vi "FFT_ADXL345.vi"() -> ()   [LabVIEW 2015]
uses:
  <vilib>/Utility/error.llb/DialogType.ctl
  <vilib>/Instr/_visa.llb/VISA Configure Serial Port (Instr).vi
panel:
  in  "Frame rate":i32
  out "FFT Graph":dbl[](graph)
  out "TIME Graph":dbl[](graph)
  out "Z":dbl
  out "Y":dbl
  out "X":dbl
  out "acceleretion(m/s^2)":cluster{"X":dbl, "Y":dbl, "Z":dbl}
  out "Waveform Chart":u32(graph)
  out "1LOOP(ms)":u32
  in  "FFT SIZE":i32
  out "DATA array":dbl[](array[numeric])
  in  "Axis":enum16{"Z", "Y", "X"}(ring)
  in  "DAC":i32
  out "DATA":string
  out "DATA LENGHT":i32
  out "Z":string
  out "Y":string
  out "X":string
  out "X(mg)":dbl format="%.2f"
  out "Y(mg)":dbl format="%.2f"
  out "Z(mg)":dbl format="%.2f"
  out "Akselerasi (mg)":dynamicdata(graph)
  in  "stop":bool
  in  "VISA RESOURCE":refnum<visa-resource-name>="COM4"
  out "millisecond timer value":u32
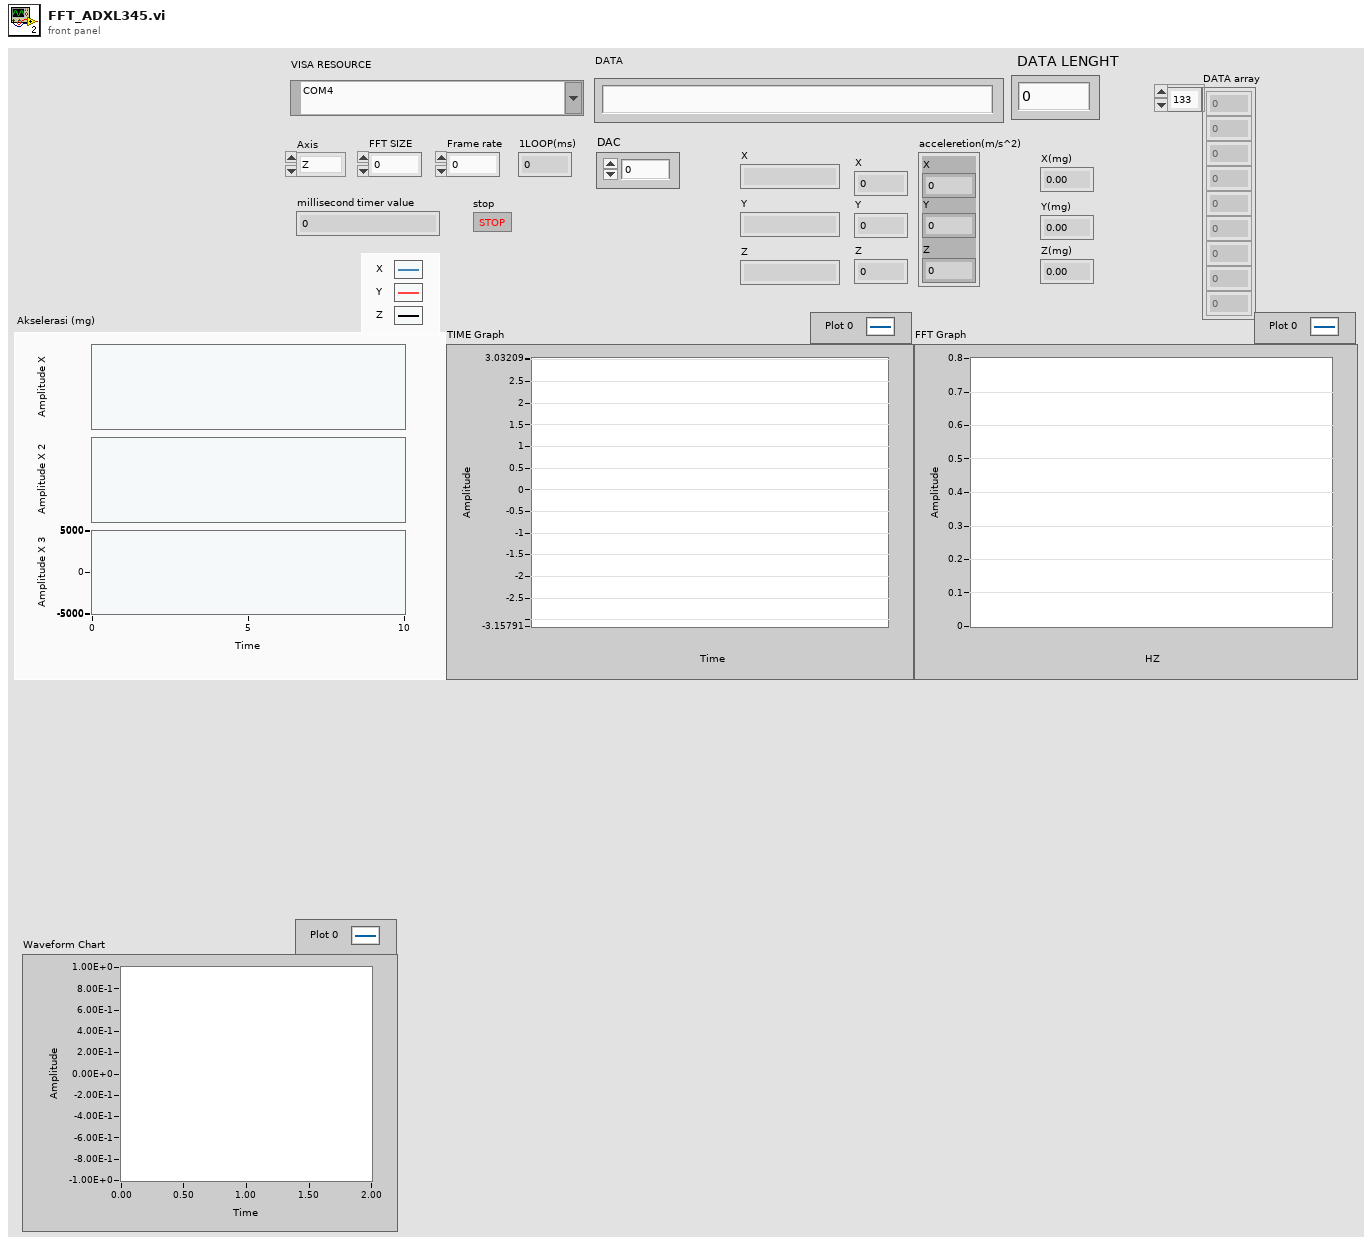
[diagram p1: front panel]
types:
  T1 = typedef "DialogType.ctl" = u16
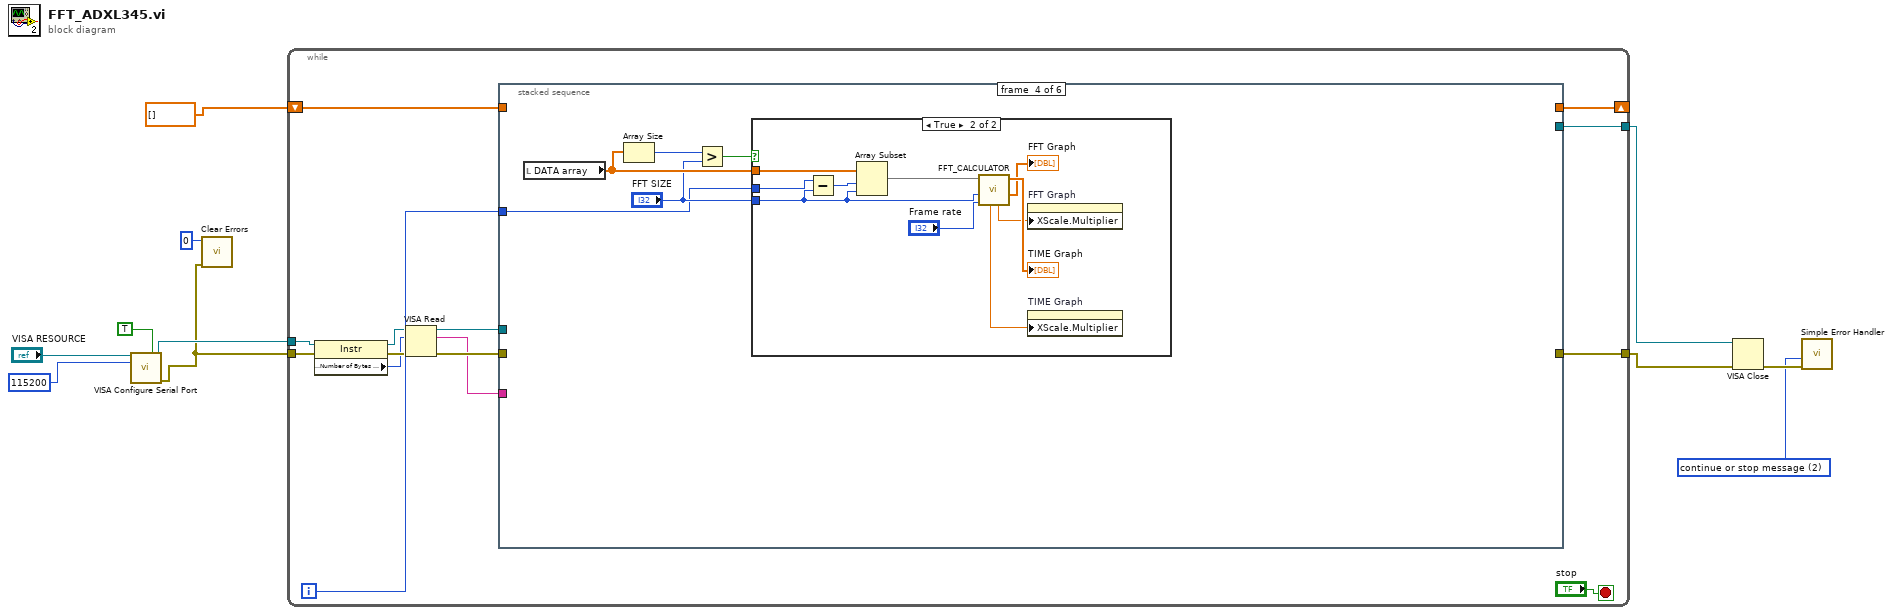
[diagram p0: block diagram]
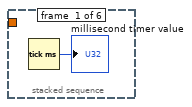
[diagram p2: hidden frame]
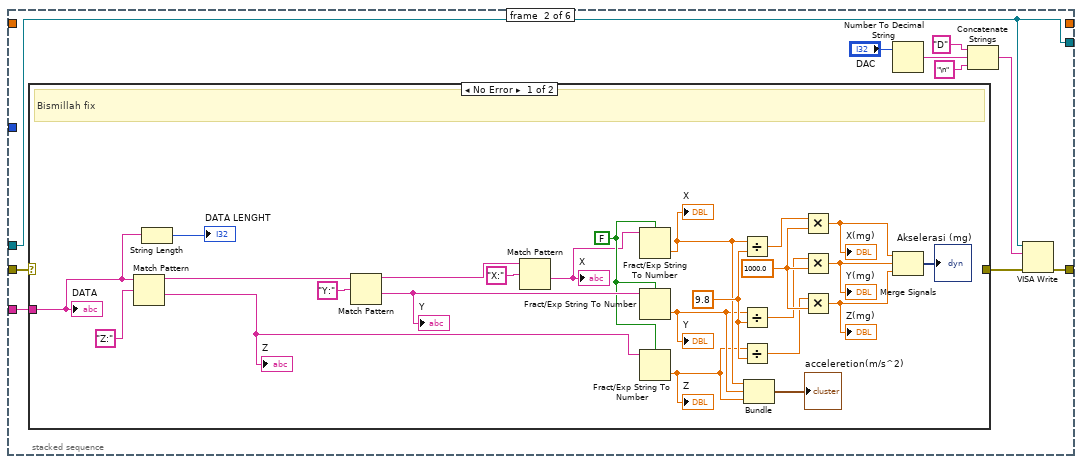
[diagram p3: hidden frame]
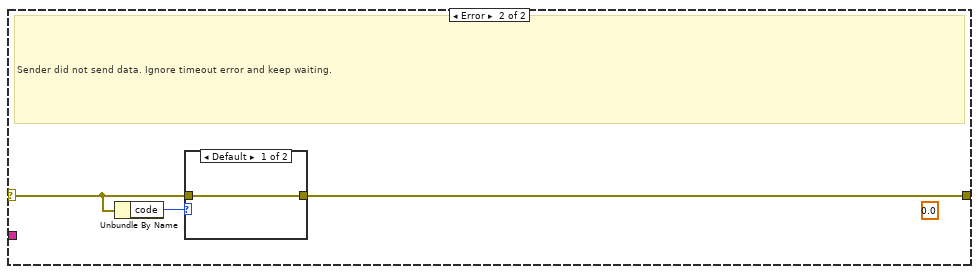
[diagram p4: hidden frame]
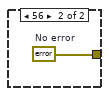
[diagram p5: hidden frame]
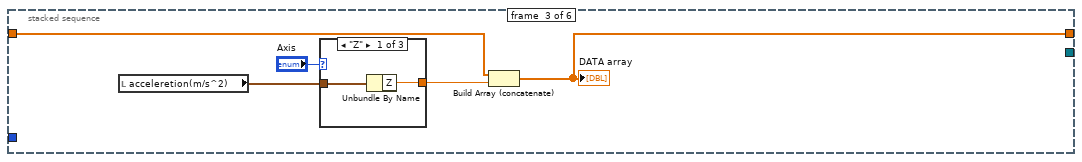
[diagram p6: hidden frame]
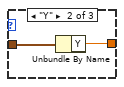
[diagram p7: hidden frame]
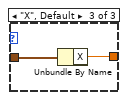
[diagram p8: hidden frame]
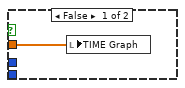
[diagram p9: hidden frame]
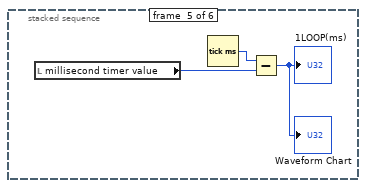
[diagram p10: hidden frame]
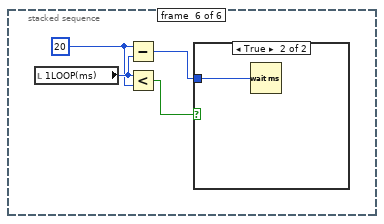
[diagram p11: hidden frame]
diagram:
  w4 = T1 2 items=["no dialog", "OK message", "continue or stop message", "OK message + warnings", "continue/stop + warnings"] ("type of dialog (OK msg:1)")
  n1 = call-poly "VISA Configure Serial Port"("VISA resource name"="VISA RESOURCE", "Enable Termination\nChar (T)"=TRUE ("Enable Termination\nChar (T)"), "baud rate (9600)"=u32 115200 ("Baud Rate")) -> ("VISA resource name out"=w7:refnum<visa-resource-name>, "error out"=w6:errorcluster)  [unwired: 11 in]
  n2 = call <vilib>:"Clear Errors.vi"("error in (no error)"=w6, "specific error code to clear (0: all)"=0) -> ()  [unwired: 4 in, 2 out]
  n3 = while {
    tunnel: w7 -> [w16]
    tunnel: w6 -> [w15]
    tunnel: [w24] -> w3
    tunnel: [w23] -> w2
    shift-right: [w21] -> _
    shift-left: dbl[] [] -> [w22]
    i -> [w20]
    stop <- "stop" stop-if-true
    n4 = property class="Instr"(reference=w16, error in=w15) -> (reference out=w19:refnum<visa-resource-name>, error out=w18:errorcluster, "Serial Settings:Number of Bytes at Serial Port"=w17:u32)
    n5 = VISA Read(VISA resource name=w19, byte count=w17, error in (no error)=w18) -> (VISA resource name out=w14:refnum<visa-resource-name>, read buffer=w12:string, error out=w13:errorcluster)  [unwired: 1 out]
    n6 = stacked-sequence {
      tunnel: [_ w30 _ _ _ _] -> w24
      tunnel: [_ w29 _ _ _ _] -> w23
      tunnel: w22 -> [_ _ w68 _ _ _]
      tunnel: [_ _ w67 _ _ _] -> w21
      tunnel: w20 -> [_ _ _ w77 _ _]
      tunnel: w14 -> [_ w29 _ _ _ _]
      tunnel: w13 -> [_ w28 _ _ _ _]
      tunnel: w12 -> [_ w27 _ _ _ _]
      frame #0 {
        n7 = Tick Count (ms)() -> (millisecond timer value=→"millisecond timer value":u32)
      }
      frame #1 {
        n8 = case shown="No Error" w28 {
          selector: w28 -> [_ w62]
          tunnel: [_ w61] -> w31
          tunnel: w27 -> [w57 _]
          frame No Error {
            w51 = 9.8
            w52 = FALSE ("use system decimal point (T)")
            w50 = 1000.0 ("y")
            # "Bismillah fix"
            n9 = Match Pattern(string=w57, regular expression="Z:") -> (before substring=w56:string, after substring=w54:string)  [unwired: 1 in, 2 out]
            "Z" <- w54
            n10 = String Length(string=w57) -> (length=→"DATA LENGHT":i32)
            n11 = Match Pattern(string=w56, regular expression="Y:") -> (before substring=w55:string, after substring=w53:string)  [unwired: 1 in, 2 out]
            "Y" <- w53
            n12 = Match Pattern(string=w55, regular expression="X:") -> (after substring=w47:string)  [unwired: 1 in, 3 out]
            "X" <- w47
            n13 = Fract/Exp String To Number(use system decimal point (T)=w52, string=w47) -> (number=w39:dbl)  [unwired: 2 in, 1 out]
            "X" <- w39
            n14 = Fract/Exp String To Number(use system decimal point (T)=w52, string=w53) -> (number=w38:dbl)  [unwired: 2 in, 1 out]
            "Y" <- w38
            n15 = Fract/Exp String To Number(use system decimal point (T)=w52, string=w54) -> (number=w37:dbl)  [unwired: 2 in, 1 out]
            "Z" <- w37
            n16 = Divide(x=w39, y=w51) -> (x/y=w42:dbl)
            n17 = Divide(x=w38, y=w51) -> (x/y=w40:dbl)
            n18 = Divide(x=w37, y=w51) -> (x/y=w41:dbl)
            n19 = Bundle(w39, w38, w37) -> (→"acceleretion(m/s^2)":cluster{dbl, dbl, dbl})  [unwired: 1 in]
            n20 = Multiply(x=w42, y=w50) -> (x*y=w46:dbl)
            "X(mg)" <- w46
            n21 = Multiply(x=w40, y=w50) -> (x*y=w45:dbl)
            "Y(mg)" <- w45
            n22 = Multiply(x=w41, y=w50) -> (x*y=w44:dbl)
            "Z(mg)" <- w44
            n23 = Merge Signals(w46, w45, w44) -> (→"Akselerasi (mg)":dynamicdata)
            "DATA" <- w57
          }
          frame Error {
            (unwired) 0.0
            # "Sender did not send data. Ignore timeout error and keep waiting."
            n24 = Unbundle By Name(w62) -> ("code"=w63:i32)
            n25 = case shown="Default" w63 {
              tunnel: w62 -> [w64 _]
              tunnel: [w64 w65] -> w61
              frame Default {
              }
              frame 56 {
                w65 = errorcluster {"status"=FALSE, "code"=0, "source"=""}  # No error
              }
            }
          }
        }
        n26 = Number To Decimal String(number="DAC") -> (decimal integer string=w32:string)  [unwired: 1 in]
        n27 = Concatenate Strings("D" ("string"), w32, "\n" ("string")) -> (w35:string)
        n28 = VISA Write(VISA resource name=w29, write buffer=w35, error in (no error)=w31) -> (error out=w30:errorcluster)  [unwired: 2 out]
      }
      frame #2 {
        n29 = local read "acceleretion(m/s^2)"() -> (w69:cluster{"X":dbl, "Y":dbl, "Z":dbl})
        n30 = case shown="\"Z\"" "Axis" {
          tunnel: w69 -> [w72 w74 w76]
          tunnel: [w71 w73 w75] -> w66
          frame "Z" {
            n31 = Unbundle By Name(w72) -> ("Z"=w71:dbl)
          }
          frame "Y" {
            n32 = Unbundle By Name(w74) -> ("Y"=w73:dbl)
          }
          frame "X", Default {
            n33 = Unbundle By Name(w76) -> ("X"=w75:dbl)
          }
        }
        n34 = Build Array (concatenate) "Build Array"(w68, w66) -> (w67:dbl[])
        "DATA array" <- w67
      }
      frame #3 {
        n35 = local read "DATA array"() -> (w79:dbl[])
        n36 = Array Size(array=w79) -> (size(s)=w81:i32)
        n37 = Greater?(x=w81, y="FFT SIZE") -> (0:w80:bool)
        n38 = case shown="True" w80 {
          tunnel: w79 -> [w82 w92]
          tunnel: "FFT SIZE" -> [_ w85]
          tunnel: w77 -> [_ w90]
          frame False {
            n39 = local write "TIME Graph"(w82) -> ()
          }
          frame True {
            n40 = Subtract(x=w90, y=w85) -> (x-y=w91:i32)
            n41 = Array Subset(array=w92, index=w91, length=w85) -> (w84:dbl[])
            n42 = call "FFT_CALCULATOR.vi"("Frame rate"="Frame rate", "FFT size"=w85, "lm"=w84) -> ("Magnitude"=→"FFT Graph":dbl[], "lm-m"=→"TIME Graph":dbl[], "df"=w86:dbl, "dt"=w87:dbl)  [unwired: 5 in]
            n43 = property on="FFT Graph" class="WFGraph (strict)"("XScale.Multiplier"=w86) -> ()  [unwired: 2 in, 2 out]
            n44 = property on="TIME Graph" class="WFGraph (strict)"("XScale.Multiplier"=w87) -> ()  [unwired: 2 in, 2 out]
          }
        }
      }
      frame #4 {
        n45 = local read "millisecond timer value"() -> (w94:u32)
        n46 = Tick Count (ms)() -> (millisecond timer value=w95:u32)
        n47 = Subtract(x=w95, y=w94) -> (x-y=→"1LOOP(ms)" →"Waveform Chart":u32)
      }
      frame #5 {
        w96 = 20 ("Sample")
        n48 = local read "1LOOP(ms)"() -> (w97:u32)
        n49 = Subtract(x=w96, y=w97) -> (x-y=w98:u32)
        n50 = Less?(x=w97, y=w96) -> (x < y?=w99:bool)
        n51 = case shown="True" w99 {
          tunnel: w98 -> [_ w100]
          frame False {
          }
          frame True {
            n52 = Wait (ms)(milliseconds to wait=w100) -> ()  [unwired: 1 out]
          }
        }
      }
    }
  }
  n53 = VISA Close(VISA resource name=w2, error in (no error)=w3) -> (error out=w5:errorcluster)
  n54 = call <vilib>:"Simple Error Handler.vi"("type of dialog (OK msg:1)"=w4, "error in (no error)"=w5) -> ()  [unwired: 3 in, 5 out]
